vi "Many Modules Example.vi"() -> ()   [LabVIEW 2017, in "Logger Examples.lvlib"]
uses:
  Logger Examples.lvlib
  Source/Composed Log/Types/Log Level.ctl
  Source/Composed Log/LoggerReference/LoggerReference.lvclass/LoggerReference.ctl
  601d143e-8928-4a3b-9174-3083e729aaa9.vi
  65753f09-765e-47a9-9fe1-17f749b2bdde.vi
  a29f9384-7d33-4f24-8d7b-0678d6b00c67.vi
  dbcf198d-a585-44a6-82a4-6996b7d4d362.vi
  Source/Composed Log/LoggerReference/Return Aggregate Queues.vi
  Source/Composed Log/LoggerReference/Add Aggregate Log.vi
  601d143e-8928-4a3b-9174-3083e729aaa9.vi/412b47dd-7504-485e-a1a1-bbc829865298.vi
  Source/Composed Log/LoggerReference/Log.vi
  65753f09-765e-47a9-9fe1-17f749b2bdde.vi/a4e2f48d-0524-4626-851f-8b9a4efcda90.vi
  a29f9384-7d33-4f24-8d7b-0678d6b00c67.vi/322d6e4f-366b-4ef2-a9ae-96b6be90c37f.vi
  dbcf198d-a585-44a6-82a4-6996b7d4d362.vi/7b8f86d1-c0dc-4143-b042-c4d0e78ce153.vi
  Source/Composed Log/LoggerReference/Send Add Sink.vi
  Source/Composed Log/LoggerReference/Remove Stale Logs.vi
  Source/String Control Sink/String Control Sink.lvclass
  C:/CS/Internal/LabVIEW/Logger/Source/Composed Log/Log Sink/Log Sink.lvclass
  Source/Composed Log/Application Logger/Launch Worker Loop.vi
  Source/Composed Log/LoggerReference/Initialize Logger Instance.vi
  Source/Composed Log/LoggerReference/LoggerReference.lvclass
  Source/Composed Log/IErrorFormat/IErrorFormat.lvclass
  Source/Composed Log/Log Sink/Log Sink.lvclass
  Source/Composed Log/Composed Log.lvlib
panel:
  out "Module 2 SubModule":string
  in  "Log Error":bool
  in  "Error Information":string
  in  "Error Code":i32
  in  "Event Level":T1(ring)
  out "Module 2":string
  out "Global Log":string
  out "Module 1":string
  in  "Data To Log":string
  in  "Source":string="User"
  in  "Log":bool
  # "Run the VI. Note how each module maintains its own log of events, and the global log captures all events. Use the 'Log' and 'Log Error' buttons to add events to the global log. See the block diagram for details."
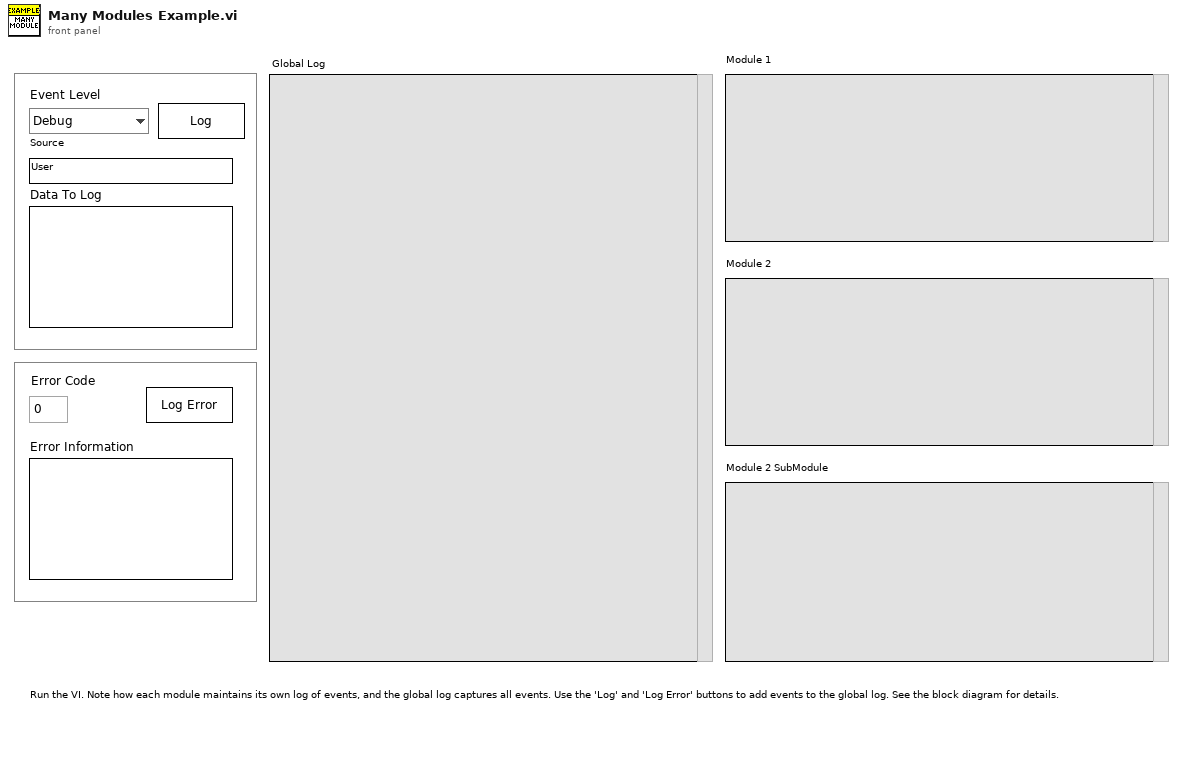
[diagram p1: front panel]
types:
  T1 = enum16{"Debug", "Info", "Warning", "Error", "Critical"}
  T2 = typedef "Composed Log.lvlib/Log Level.ctl" = enum16{"Debug", "Info", "Warning", "Error", "Critical"}
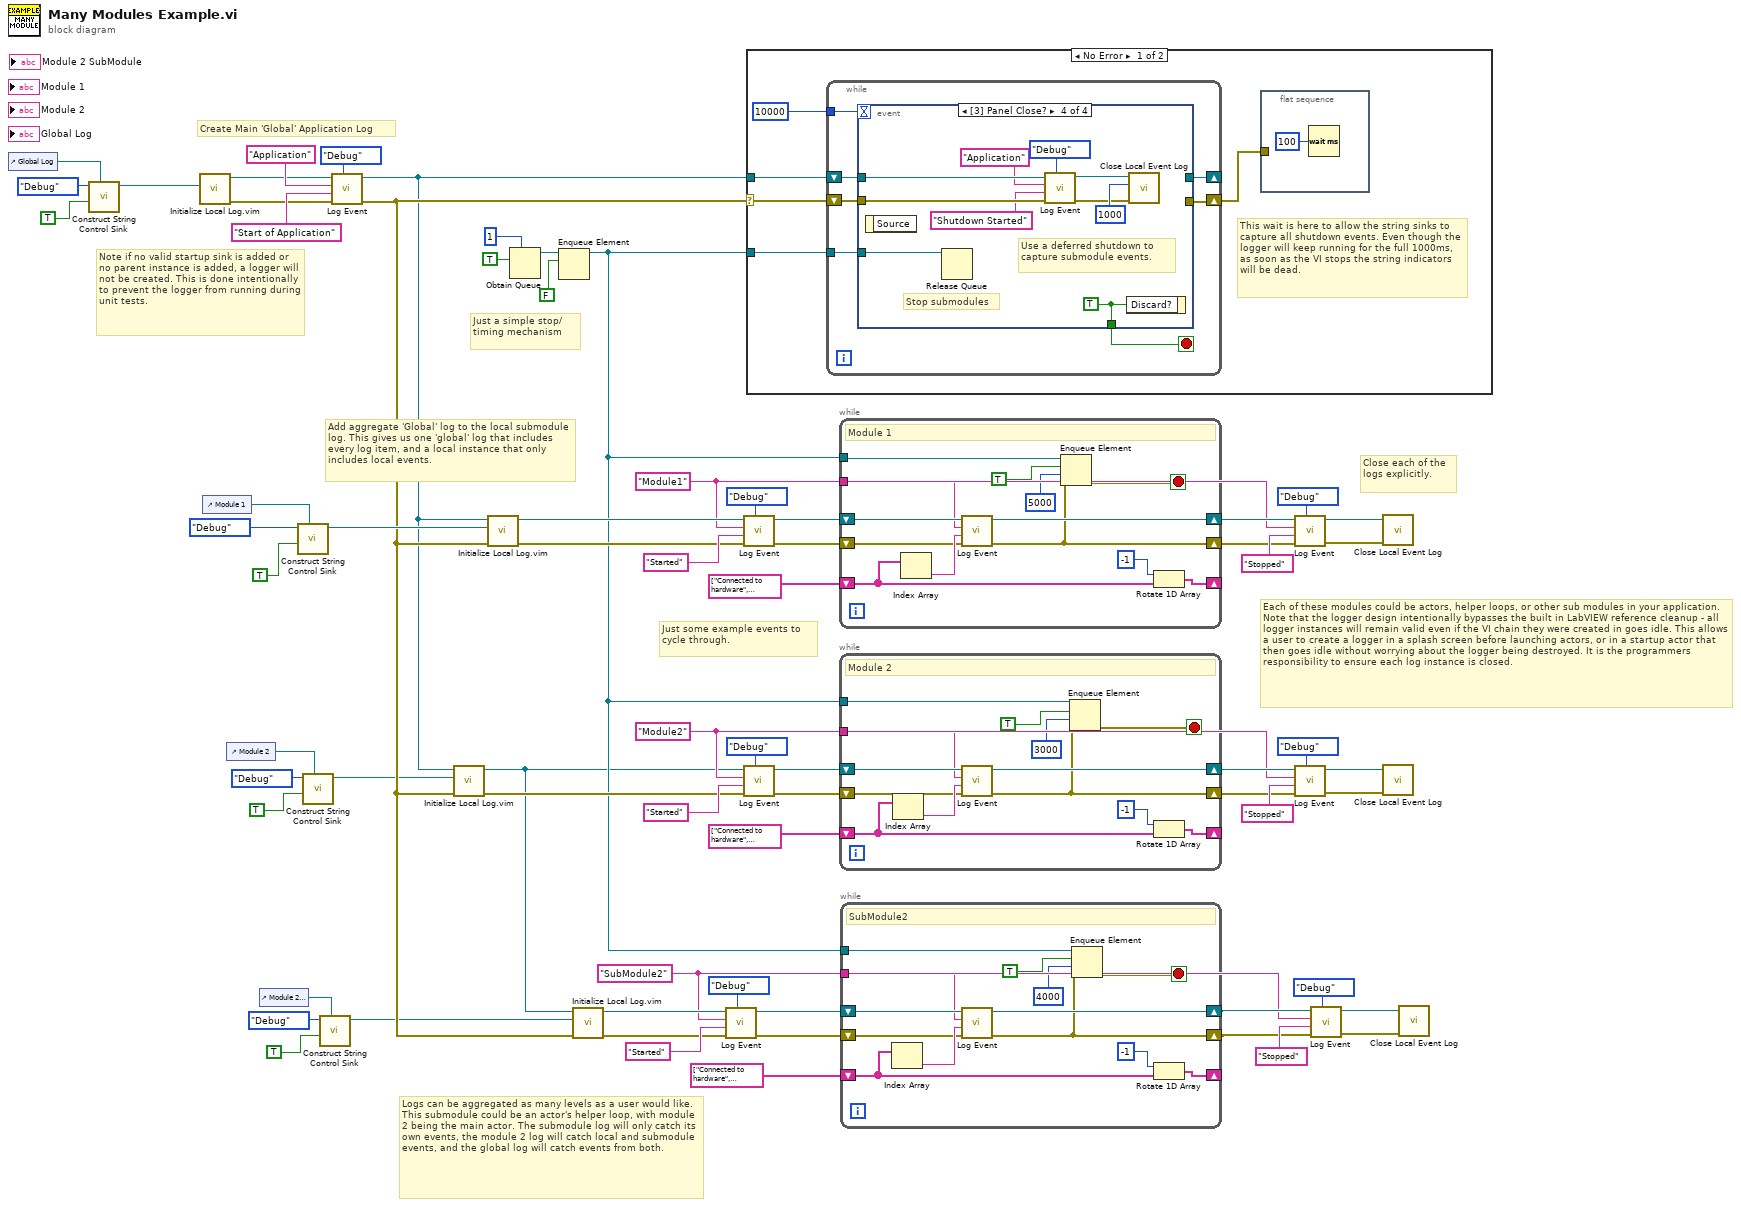
[diagram p0: block diagram]
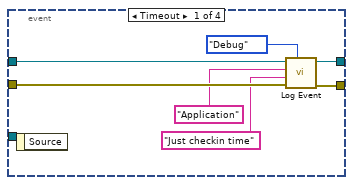
[diagram p2: hidden frame]
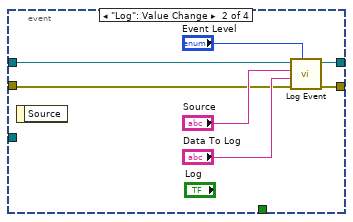
[diagram p3: hidden frame]
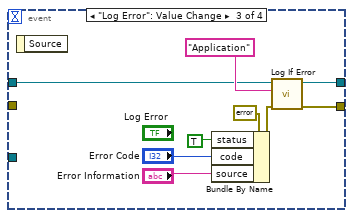
[diagram p4: hidden frame]
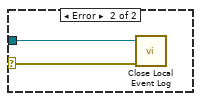
[diagram p5: hidden frame]
diagram:
  w14 = "SubModule2" ("Data To Log")
  w34 = "Module2" ("Data To Log")
  w50 = "Module1" ("Data To Log")
  # "Note if no valid startup sink is added or no parent instance is added, a logger will not be created. This is done intentionally to prevent the logger from running during unit tests."
  # "Logs can be aggregated as many levels as a user would like. This submodule could be an actor's helper loop, with module 2 being the main actor. The submodule log will only catch its own events, the module 2 log will catch local and submodule events, and the global log will catch events from both."
  # "Each of these modules could be actors, helper loops, or other sub modules in your application. Note that the logger design intentionally bypasses the built in LabVIEW reference cleanup - all logger instances will remain valid even if the VI chain they were created in goes idle. This allows a user to create a logger in a splash screen before launching actors, or in a startup actor that then goes idle without worrying about the logger being destroyed. It is the programmers responsibility to ensure each log instance is closed."
  # "Just some example events to cycle through."
  # "Add aggregate 'Global' log to the local submodule log. This gives us one 'global' log that includes every log item, and a local instance that only includes local events."
  # "Create Main 'Global' Application Log"
  # "Just a simple stop/timing mechanism"
  # "Close each of the logs explicitly."
  n1 = control-ref of="Global Log"() -> (w66:refnum<vi>)
  n2 = call "Construct String Control Sink.vi"("Str Refnum"=w66, "AutoScroll?(F)"=TRUE, "LogLevel"=Log_Level."Debug") -> ("String Control Sink out"=w60:refnum<class "String Control Sink.lvclass">)  [unwired: 8 in]
  n3 = call "Initialize Local Log.vim"("Startup Sink(s)"=w60) -> ("error out"=w7:errorcluster, "Log Instance Reference"=w6:refnum<class "LoggerReference.lvclass">)  [unwired: 8 in, 1 out]
  n4 = control-ref of="Module 1"() -> (w68:refnum<vi>)
  n5 = control-ref of="Module 2"() -> (w62:refnum<vi>)
  n6 = control-ref of="Module 2 SubModule"() -> (w11:refnum<vi>)
  n7 = call "Construct String Control Sink.vi"("Str Refnum"=w68, "AutoScroll?(F)"=TRUE, "LogLevel"=Log_Level."Debug") -> ("String Control Sink out"=w61:refnum<class "String Control Sink.lvclass">)  [unwired: 8 in]
  n8 = call "Construct String Control Sink.vi"("Str Refnum"=w62, "AutoScroll?(F)"=TRUE, "LogLevel"=Log_Level."Debug") -> ("String Control Sink out"=w3:refnum<class "String Control Sink.lvclass">)  [unwired: 8 in]
  n9 = call "Construct String Control Sink.vi"("Str Refnum"=w11, "AutoScroll?(F)"=TRUE, "LogLevel"=Log_Level."Debug") -> ("String Control Sink out"=w4:refnum<class "String Control Sink.lvclass">)  [unwired: 8 in]
  n10 = call "Log Event.vi"("Event Level"=Log_Level."Debug", "error in (no error)"=w7, "Data To Log"="Start of Application", "SourceID"="Application", "Log Instance"=w6) -> ("error out"=w5:errorcluster, "Log Instance Out"=w2:refnum<class "LoggerReference.lvclass">)  [unwired: 5 in]
  n11 = call "Initialize Local Log.vim"("error in (no error)"=w5, "Startup Sink(s)"=w3, "Parent Log Reference"=w2) -> ("error out"=w29:errorcluster, "Log Instance Reference"=w1:refnum<class "LoggerReference.lvclass">)  [unwired: 6 in, 1 out]
  n12 = call "Initialize Local Log.vim"("error in (no error)"=w5, "Startup Sink(s)"=w61, "Parent Log Reference"=w2) -> ("error out"=w51:errorcluster, "Log Instance Reference"=w53:refnum<class "LoggerReference.lvclass">)  [unwired: 6 in, 1 out]
  n13 = Obtain Queue(max queue size (-1, unlimited)=1, element data type=TRUE) -> (queue out=w46:refnum<queue>)  [unwired: 3 in, 2 out]
  n14 = Enqueue Element(queue=w46, element=FALSE) -> (queue out=w21:refnum<queue>)  [unwired: 2 in, 2 out]
  n15 = call "Initialize Local Log.vim"("error in (no error)"=w5, "Startup Sink(s)"=w4, "Parent Log Reference"=w1) -> ("error out"=w24:errorcluster, "Log Instance Reference"=w23:refnum<class "LoggerReference.lvclass">)  [unwired: 6 in, 1 out]
  n16 = call "Log Event.vi"("Event Level"=Log_Level."Debug", "error in (no error)"=w24, "Data To Log"="Started", "SourceID"=w14, "Log Instance"=w23) -> ("error out"=w26:errorcluster, "Log Instance Out"=w25:refnum<class "LoggerReference.lvclass">)  [unwired: 5 in]
  n17 = call "Log Event.vi"("Event Level"=Log_Level."Debug", "error in (no error)"=w51, "Data To Log"="Started", "SourceID"=w50, "Log Instance"=w53) -> ("error out"=w49:errorcluster, "Log Instance Out"=w52:refnum<class "LoggerReference.lvclass">)  [unwired: 5 in]
  n18 = call "Log Event.vi"("Event Level"=Log_Level."Debug", "error in (no error)"=w29, "Data To Log"="Started", "SourceID"=w34, "Log Instance"=w1) -> ("error out"=w33:errorcluster, "Log Instance Out"=w35:refnum<class "LoggerReference.lvclass">)  [unwired: 5 in]
  n19 = case shown="No Error" w5 {
    selector: w5 -> [w73 w117]
    tunnel: w2 -> [w75 w118]
    tunnel: w21 -> [w74 _]
    frame No Error {
      # "This wait is here to allow the string sinks to capture all shutdown events. Even though the logger will keep running for the full 1000ms, as soon as the VI stops the string indicators will be dead."
      n20 = while {
        shift-right: [w81] -> _
        shift-left: w75 -> [w82]
        tunnel: w74 -> [w80]
        shift-right: [w78] -> w71
        shift-left: w73 -> [w79]
        tunnel: 10000 -> [w77]
        stop <- w83 stop-if-true
        n21 = event shown="[3] Panel Close?" {
          selector: _ -> [_ _ _ _]
          dyn-events: _ -> [_ _ _ _]
          timeout: w77 -> [_ _ _ _]
          tunnel: [_ _ _ w116] -> w83
          tunnel: w82 -> [w87 w94 w100 w112]
          tunnel: [w88 w92 w98 _] -> w81
          tunnel: w80 -> [_ _ _ w115]
          tunnel: w79 -> [w90 w91 _ w113]
          tunnel: [w89 w93 w99 _] -> w78
          event Timeout {
            n22 = event-data() -> ()  [unwired: 1 in, 1 out]
            n23 = call "Log Event.vi"("Event Level"=Log_Level."Debug", "error in (no error)"=w90, "Data To Log"="Just checkin time", "SourceID"="Application", "Log Instance"=w87) -> ("error out"=w89:errorcluster, "Log Instance Out"=w88:refnum<class "LoggerReference.lvclass">)  [unwired: 5 in]
          }
          event "Log": Value Change {
            n24 = event-data() -> ()  [unwired: 1 in, 1 out]
            n25 = call "Log Event.vi"("Event Level"="Event Level", "error in (no error)"=w91, "Data To Log"="Data To Log", "SourceID"="Source", "Log Instance"=w94) -> ("error out"=w93:errorcluster, "Log Instance Out"=w92:refnum<class "LoggerReference.lvclass">)  [unwired: 5 in]
          }
          event "Log Error": Value Change {
            n26 = event-data() -> ()  [unwired: 1 in, 1 out]
            n27 = Bundle By Name(cluster=errorcluster {"status"=FALSE, "code"=0, "source"=""} ("Error In"), "status"=TRUE, "code"="Error Code", "source"="Error Information") -> (w104:errorcluster)
            n28 = call "Log If Error.vi"("Error In"=w104, "SourceID"="Application" ("Source"), "Log Instance"=w100) -> ("error out"=w99:errorcluster, "Log Instance Out"=w98:refnum<class "LoggerReference.lvclass">)  [unwired: 7 in]
          }
          event Panel Close? {
            w116 = TRUE ("Discard?")
            # "Use a deferred shutdown to capture submodule events."
            # "Stop submodules"
            n29 = event-data() -> ()  [unwired: 1 in, 1 out]
            n30 = Release Queue(queue=w115) -> ()  [unwired: 2 in, 3 out]
            n31 = call "Log Event.vi"("Event Level"=Log_Level."Debug", "error in (no error)"=w113, "Data To Log"="Shutdown Started", "SourceID"="Application", "Log Instance"=w112) -> ("error out"=w111:errorcluster, "Log Instance Out"=w110:refnum<class "LoggerReference.lvclass">)  [unwired: 5 in]
            n32 = event-data("Discard?"=w116) -> ()  [unwired: 1 in, 1 out]
            n33 = call "Close Local Event Log.vi"("error in (no error)"=w111, "Deferred Close Time (0 ms)"=u32 1000, "Log Instance"=w110) -> ()  [unwired: 8 in, 1 out]
          }
        }
      }
      n34 = flat-sequence {
        tunnel: w71 -> [_]
        frame #0 {
          n35 = Wait (ms)(milliseconds to wait=u32 100) -> ()  [unwired: 1 out]
        }
      }
    }
    frame Error {
      n36 = call "Close Local Event Log.vi"("error in (no error)"=w117, "Log Instance"=w118) -> ()  [unwired: 9 in, 1 out]
    }
  }
  n37 = while {
    shift-right: [w129] -> w59
    shift-left: w52 -> [w131]
    tunnel: w50 -> [w130]
    shift-right: [w119] -> w42
    shift-left: w49 -> [w120]
    tunnel: w21 -> [w128]
    shift-right: [w124] -> _
    shift-left: string[] ["Connected to hardware", "Collected some data", "Disconnected from hardware.", "Went to idle model", "Received data collection request"] -> [w126]
    stop <- w121 stop-if-true
    # "Module 1"
    n38 = Index Array(array=w126) -> (element=w125:string)  [unwired: 1 in]
    n39 = call "Log Event.vi"("error in (no error)"=w120, "Data To Log"=w125, "SourceID"=w130, "Log Instance"=w131) -> ("error out"=w119:errorcluster, "Log Instance Out"=w129:refnum<class "LoggerReference.lvclass">)  [unwired: 6 in]
    n40 = Enqueue Element(queue=w128, element=TRUE, timeout in ms (-1)=5000, error in (no error)=w119) -> (error out=w121:errorcluster)  [unwired: 2 out]
    n41 = Rotate 1D Array(1:w126, 2:-1 ("n")) -> (0:w124:string[])
  }
  n42 = while {
    shift-right: [w142] -> w41
    shift-left: w35 -> [w144]
    tunnel: w34 -> [w143]
    shift-right: [w132] -> w30
    shift-left: w33 -> [w134]
    tunnel: w21 -> [w141]
    shift-right: [w137] -> _
    shift-left: string[] ["Connected to hardware", "Collected some data", "Disconnected from hardware.", "Went to idle model", "Received data collection request"] -> [w139]
    stop <- w133 stop-if-true
    # "Module 2"
    n43 = Index Array(array=w139) -> (element=w138:string)  [unwired: 1 in]
    n44 = call "Log Event.vi"("error in (no error)"=w134, "Data To Log"=w138, "SourceID"=w143, "Log Instance"=w144) -> ("error out"=w132:errorcluster, "Log Instance Out"=w142:refnum<class "LoggerReference.lvclass">)  [unwired: 6 in]
    n45 = Enqueue Element(queue=w141, element=TRUE, timeout in ms (-1)=3000, error in (no error)=w132) -> (error out=w133:errorcluster)  [unwired: 2 out]
    n46 = Rotate 1D Array(1:w139, 2:-1 ("n")) -> (0:w137:string[])
  }
  n47 = while {
    shift-right: [w155] -> w15
    shift-left: w25 -> [w157]
    tunnel: w14 -> [w156]
    shift-right: [w145] -> w16
    shift-left: w26 -> [w147]
    tunnel: w21 -> [w154]
    shift-right: [w150] -> _
    shift-left: string[] ["Connected to hardware", "Collected some data", "Disconnected from hardware.", "Went to idle model", "Received data collection request"] -> [w152]
    stop <- w146 stop-if-true
    # "SubModule2"
    n48 = Index Array(array=w152) -> (element=w151:string)  [unwired: 1 in]
    n49 = call "Log Event.vi"("error in (no error)"=w147, "Data To Log"=w151, "SourceID"=w156, "Log Instance"=w157) -> ("error out"=w145:errorcluster, "Log Instance Out"=w155:refnum<class "LoggerReference.lvclass">)  [unwired: 6 in]
    n50 = Enqueue Element(queue=w154, element=TRUE, timeout in ms (-1)=4000, error in (no error)=w145) -> (error out=w146:errorcluster)  [unwired: 2 out]
    n51 = Rotate 1D Array(1:w152, 2:-1 ("n")) -> (0:w150:string[])
  }
  n52 = call "Log Event.vi"("Event Level"=Log_Level."Debug", "error in (no error)"=w42, "Data To Log"="Stopped", "SourceID"=w50, "Log Instance"=w59) -> ("error out"=w43:errorcluster, "Log Instance Out"=w58:refnum<class "LoggerReference.lvclass">)  [unwired: 5 in]
  n53 = call "Log Event.vi"("Event Level"=Log_Level."Debug", "error in (no error)"=w30, "Data To Log"="Stopped", "SourceID"=w34, "Log Instance"=w41) -> ("error out"=w31:errorcluster, "Log Instance Out"=w40:refnum<class "LoggerReference.lvclass">)  [unwired: 5 in]
  n54 = call "Log Event.vi"("Event Level"=Log_Level."Debug", "error in (no error)"=w16, "Data To Log"="Stopped", "SourceID"=w14, "Log Instance"=w15) -> ("error out"=w17:errorcluster, "Log Instance Out"=w20:refnum<class "LoggerReference.lvclass">)  [unwired: 5 in]
  n55 = call "Close Local Event Log.vi"("error in (no error)"=w43, "Log Instance"=w58) -> ()  [unwired: 9 in, 1 out]
  n56 = call "Close Local Event Log.vi"("error in (no error)"=w31, "Log Instance"=w40) -> ()  [unwired: 9 in, 1 out]
  n57 = call "Close Local Event Log.vi"("error in (no error)"=w17, "Log Instance"=w20) -> ()  [unwired: 9 in, 1 out]
